vi "FindEnumInProject.vi"(8 "error in (no error)":errorcluster, 10 "Name":string) -> (0 "error out":errorcluster, 1 "Found":bool, 2 "ProjectItem Refnum":refnum<vi>)   [LabVIEW 2013, in "GenLVOOP.lvclass"]
uses:
  GenLVOOP.lvclass
  ProjectHandler/RefNums.vi
  ProjectHandler.lvlib
panel:
  out "Type String":string
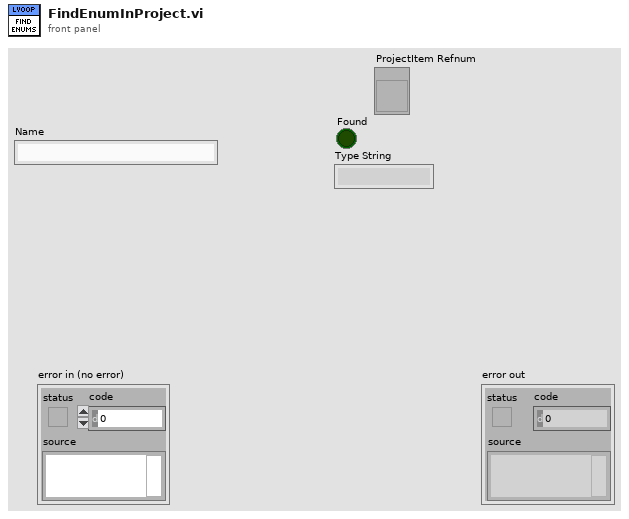
[diagram p1: front panel]
types:
  T1 = cluster{"App":refnum<vi>, "Project":refnum<vi>, "My Computer":refnum<vi>}
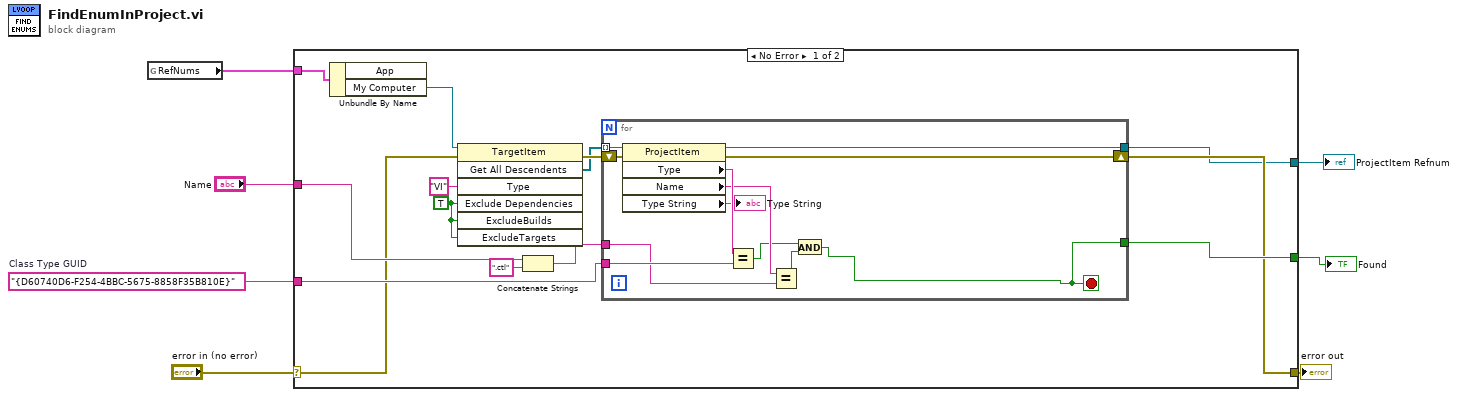
[diagram p0: block diagram]
diagram:
  w4 = "{D60740D6-F254-4BBC-5675-8858F35B810E}"  # Class Type GUID
  n1 = global read "RefNums.vi" "RefNums"() -> (w5:T1)
  n2 = case shown="No Error" "error in (no error)" {
    selector: "error in (no error)" -> [w12 w34]
    tunnel: [w15 w34] -> w6
    tunnel: w5 -> [w21 _]
    tunnel: w4 -> [w20 _]
    tunnel: [w19 _] -> w3
    tunnel: "Name" -> [w16 _]
    tunnel: [w14 _] -> w1
    frame No Error {
      w8 = TRUE ("ExcludeDependencies")
      n3 = Unbundle By Name(w21) -> ("My Computer"=w13:refnum<vi>)  [unwired: 1 out]
      n4 = invoke class="TargetItem" method="Get All Descendents"(reference=w13, error in=w12, "Type"="VI", "Exclude Dependencies"=w8, "ExcludeBuilds"=w8, "ExcludeTargets"=w8) -> (error out=w11:errorcluster, "All Descendents"=w9:refnum<vi>[])  [unwired: 1 in, 5 out]
      n5 = Concatenate Strings(w16, ".ctl" ("string")) -> (w18:string)
      n6 = for {
        tunnel: w9 -> [w31] mode=indexing
        tunnel: w20 -> [w32]
        tunnel: w18 -> [w29]
        tunnel: [w26] -> w19
        shift-right: [w24] -> w15
        shift-left: w11 -> [w25]
        tunnel: [w23] -> w14
        stop <- w26 stop-if-true
        n7 = property class="ProjectItem"(reference=w31, error in=w25) -> (reference out=w23:refnum<vi>, error out=w24:errorcluster, "Type"=w33:string, "Name"=w30:string, "Type String"=→"Type String":string)
        n8 = Equal?(x=w33, y=w32) -> (x = y?=w27:bool)
        n9 = Equal?(x=w30, y=w29) -> (x = y?=w28:bool)
        n10 = And(x=w27, y=w28) -> (x .and. y?=w26:bool)
      }
    }
    frame Error {
    }
  }
  "error out" <- w6
  "Found" <- w3
  "ProjectItem Refnum" <- w1
